vi "MSFET202_Temp_CalibCalc.vi"(11 "\"VTherm\"":dbl=0.8611887382361767) -> (2 "Temperature (C)":dbl=24.4655047055293)   [LabVIEW 2018]
panel:
  in  "calVoltage":dbl=0.8612
  in  "calTemp":dbl=22.71
  # "MSFET 3332 202x"
  # "INPUTS"
  # "OUTPUTS"
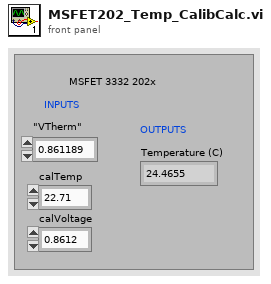
[diagram p1: front panel]
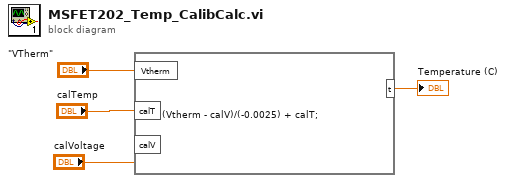
[diagram p0: block diagram]
diagram:
  n1 = formula code="t = (Vtherm - calV)/(-0.0025) + calT;"("Vtherm"="\"VTherm\"", "calT"="calTemp", "calV"="calVoltage") -> ("t"=→"Temperature (C)":dbl)
